vi "Values.vi"(8 "error in (no error)":errorcluster, 11 "StringMap in":refnum<class "StringMap.lvclass">) -> (0 "error out":errorcluster, 1 "Values":string[](array[string]), 3 "StringMap out":refnum<class "StringMap.lvclass">)   [LabVIEW 2013, in "LapDog.Collections.v_.Maps.lvlib" / "StringMap.lvclass"]
doc: "Returns a copy of all values in the map."
uses:
  StringMap.lvclass
  LapDog.Collections.Common/String/String.lvclass
  ObjectMap/ObjectMap.lvclass
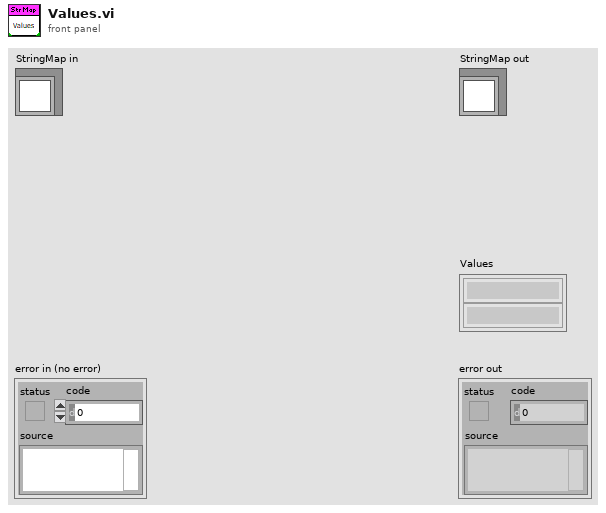
[diagram p1: front panel]
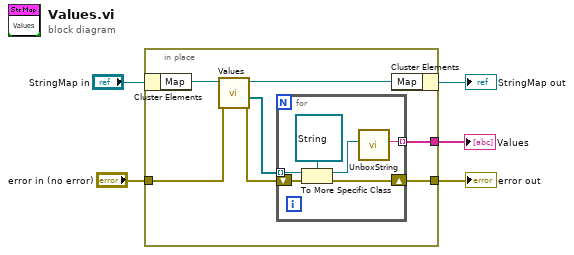
[diagram p0: block diagram]
diagram:
  n1 = in-place {
    in-place-border: "error in (no error)" -> [w10]
    in-place-border: [w7] -> w2
    in-place-border: [w6] -> w1
    n2 = in-place-cluster #1("StringMap in") -> ("Map"=w12:refnum<class "ObjectMap.lvclass">)
    n3 = call-dynamic "Values.vi"("error in (no error)"=w10, "Map in"=w12) -> ("error out"=w8:errorcluster, "Values"=w9:refnum<class>[], "Map out"=w11:refnum<class "ObjectMap.lvclass">)  [unwired: 7 in]
    n4 = for {
      tunnel: w9 -> [w18] mode=indexing
      shift-right: [w16] -> w7
      shift-left: w8 -> [w17]
      tunnel: [w13] -> w6 mode=indexing
      n5 = To More Specific Class(target class=refnum<class "String.lvclass"> refnum ("LapDog.Collections.v0.Common.lvlib:String.lvclass"), reference=w18, error in=w17) -> (specific class reference=w14:refnum<class "String.lvclass">, error out=w16:errorcluster)
      n6 = call "UnboxString.vi"("String in"=w14) -> ("String"=w13:string)  [unwired: 10 in]
    }
    n7 = in-place-cluster #1("Map"=w11) -> (→"StringMap out":refnum<class "StringMap.lvclass">)
  }
  "error out" <- w2
  "Values" <- w1
